vi "Clamp.vi"(8 "error in (no error)":errorcluster, 11 "Instrument.VRM in":refnum<class "Instrument.OxfordVRM.lvclass">) -> (0 "error out":errorcluster, 2 "Response":string, 3 "Instrument.VRM out":refnum<class "Instrument.OxfordVRM.lvclass">)   [LabVIEW 2019, in "Instrument.OxfordVRM.lvclass"]
uses:
  Instrument.OxfordVRM.lvclass
  Typedefs/Instrument.VRM.protectedCommands-enum.ctl
  6cf589e9-cbef-4283-8e70-3f344f377440.vi
  6cf589e9-cbef-4283-8e70-3f344f377440.vi/4bc8cd6b-94f6-4c5e-9207-8717120dfe1b.vi
  6cf589e9-cbef-4283-8e70-3f344f377440.vi/c4ec101b-6ff3-4c4f-971d-2ec602f2dadd.vi
  <vilib>/Utility/Data Type/Get Type Information.vi
  <vilib>/JDP Science/JSONtext/JSON text to Variant.vi
  <vilib>/JDP Science/JSONtext/LVClass Serializer/JSONtext LVClass Serializer.lvclass
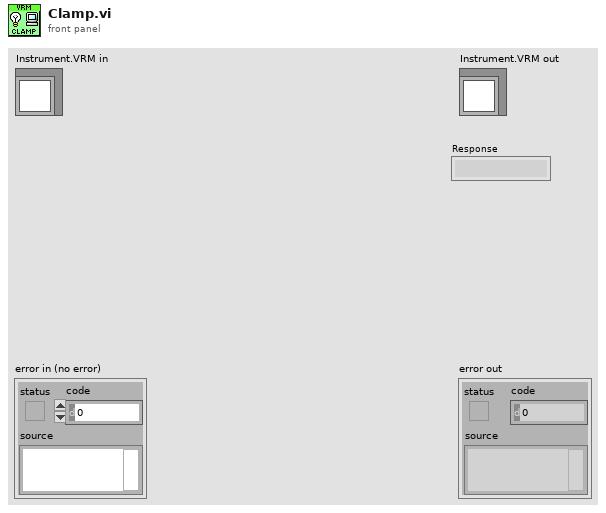
[diagram p1: front panel]
types:
  T1 = typedef "Instrument.OxfordVRM.lvclass/Instrument.VRM.protectedCommands-enum.ctl" = enum16{"Hold", "RampToSet", "RampToZero", "Clamp", "SetTarget", "GetStatus", "GetTarget", "GetField"}
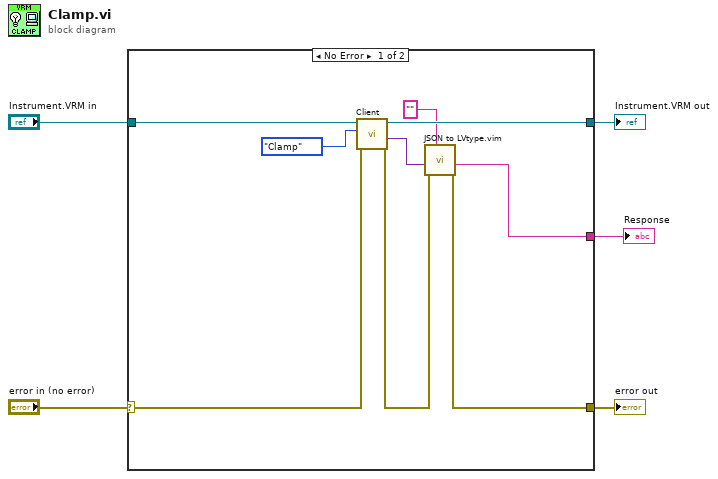
[diagram p0: block diagram]
diagram:
  n1 = case shown="No Error" "error in (no error)" {
    selector: "error in (no error)" -> [w13 w16]
    tunnel: [w11 w16] -> w4
    tunnel: [w12 w15] -> w2
    tunnel: "Instrument.VRM in" -> [w14 w15]
    tunnel: [w10 _] -> w1
    frame No Error {
      n2 = call-dynamic "Client.vi"("error in (no error)"=w13, "Command in"=Instrument.VRM.protectedCommands-enum."Clamp" ("protectedCommands"), "Instrument in"=w14) -> ("error out"=w7:errorcluster, "Data out"=w8:variant, "Instrument out"=w12:refnum<class "Instrument.OxfordVRM.lvclass">)  [unwired: 5 in, 1 out]
      n3 = call "JSON to LVtype.vim"("type"="", "error in (no error)"=w7, "JSON Data in"=w8) -> ("error out"=w11:errorcluster, "Data out"=w10:string)  [unwired: 7 in]
    }
    frame Error {
    }
  }
  "error out" <- w4
  "Instrument.VRM out" <- w2
  "Response" <- w1
